vi "Tank Drive.vi"() -> ()   [LabVIEW 2012]
doc: "Tank Drive Example\n\nThis example shows how to implement tank drive and uses two joysticks for input."
uses:
  <vilib>/Rock Robotics/SystemInterfaces/DIO/FPGA_DIOPWMChannel.ctl
  <vilib>/Rock Robotics/WPI/Joystick/WPI_JoystickDeviceEnum.ctl
  <vilib>/Rock Robotics/WPI/Joystick/WPI_JoystickAxis.ctl
  <vilib>/Rock Robotics/WPI/RobotDrive/WPI_RobotDriveOpen2MotorWithJaguar.vi
panel:
  in  "RightStick":T1=enum."USB 2"
  in  "LeftStick":T1
  in  "Left Motor (PWM channel)":T2
  in  "Right Motor (PWM channel)":T2=enum."PWM 2"
  in  "stop":bool
  # "Set these inputs before running."
  # "Wiring Diagram for Digital Sidecar connected to an NI 9403 in slot 4"
  # "Digital Sidecar"
  # "Power\nTerminals"
  # "Motor\nTerminals"
  # "PWM cable"
  # "This shows wiring for a Luminary Micro Jaguar speed controller.  The wiring is similar for a Victor speed controller.  For a Victor, you must also select the appropriate instance of the Motor Open VI on the diagram.  This is only the wiring for the Left Motor.  The Right Motor would be similarly wired to PWM Channel 2."
  # "PWR"
  # "SIG"
  # "(-)"
  # "+V"
  # "10"
  # "9"
  # "8"
  # "7"
  # "6"
  # "5"
  # "4"
  # "3"
  # "2"
  # "1"
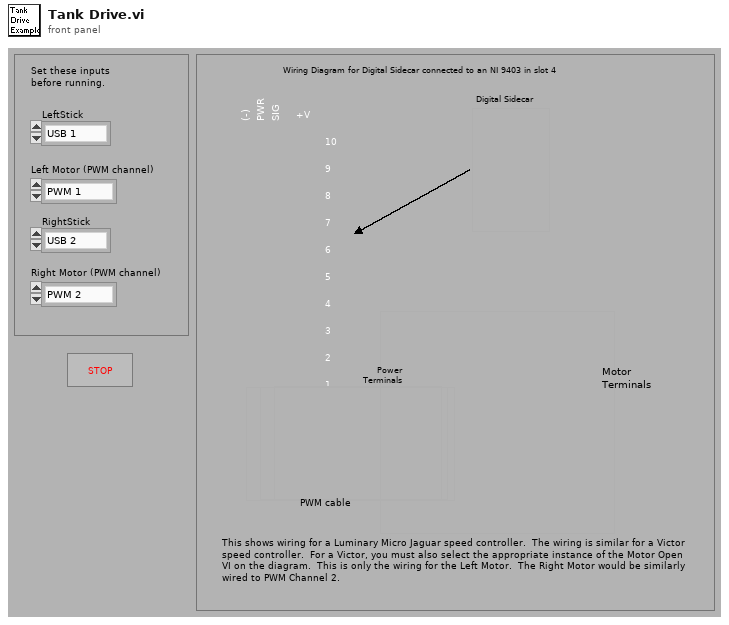
[diagram p1: front panel]
types:
  T1 = typedef "WPI_JoystickDeviceEnum.ctl" = enum16{"USB 1", "USB 2", "USB 3", "USB 4", "Kinect 1", "Kinect 2"}
  T2 = typedef "FPGA_DIOPWMChannel.ctl" = enum8{"PWM 1", "PWM 2", "PWM 3", "PWM 4", "PWM 5", "PWM 6", "PWM 7", "PWM 8", "PWM 9", "PWM 10", "Invalid"}
  T3 = typedef "WPI_JoystickDevRef.ctl" = cluster{"Device":T1}
  T4 = typedef "WPI_RobotDriveDevRef.ctl" = cluster{"DevStatus":errorcluster, "Motors[]":T5[], "Square Inputs":bool, "Max Output":dbl, "Isochronous":bool}
  T5 = typedef "WPI_MotorControlDeviceRef.ctl" = cluster{"DeviceStatus":errorcluster, "Type":enum16{"PWM", "CAN"}, "PWM":cluster{"Digital Module":T6, "PWM Channel":T2, "DeadBand":T7}, "CAN":cluster{"Device Number":u8, "Control Mode":T8, "Semaphore":T9, "Max Vout":dbl}, "Invert":bool, "TransformRef":T10, "InvTransformRef":T10}
  T6 = typedef "FPGA_TypedefDigitalModule.ctl" = enum16{"Digital Module 1", "Digital Module 2"}
  T7 = typedef "WPI_PWMDeadband.ctl" = cluster{"Name":string, "maxPositivePwm":i32, "minPositivePwm":i32, "centerPwm":i32, "maxNegativePwm":i32, "minNegativePwm":i32, "angularRange":u16}
  T8 = typedef "WPI_CANJaguar_ControlMode.ctl" = enum8{"Percent VBus", "Current", "Speed", "Position", "Voltage"}
  T9 = typedef "Semaphore RefNum" = refnum<k1>
  T10 = typedef "WPI_PWMTransform_ConPane.ctl" = refnum<vi>
  T11 = typedef "WPI_JoystickAxis.ctl" = enum16{"Axis 1", "Axis 2", "Axis 3", "Axis 4", "Axis 5", "Axis 6"}
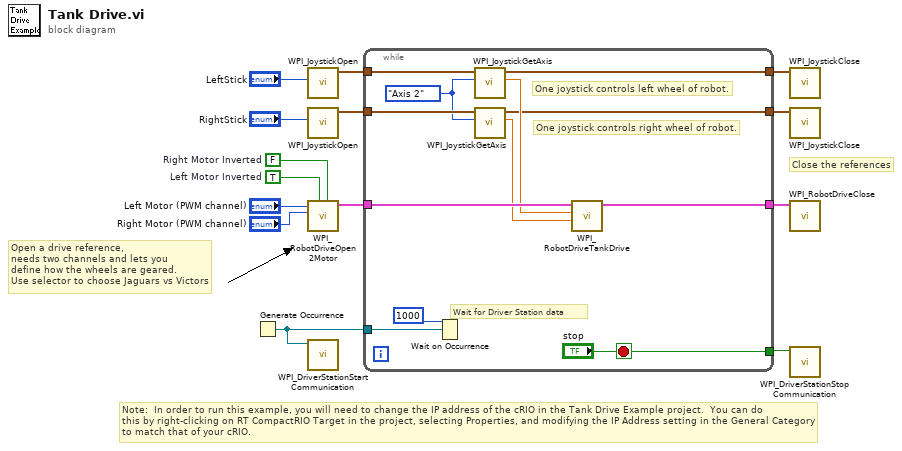
[diagram p0: block diagram]
diagram:
  w7 = FALSE  # Right Motor Inverted
  w8 = TRUE  # Left Motor Inverted
  # "Note:  In order to run this example, you will need to change the IP address of the cRIO in the Tank Drive Example project.  You can do\nthis by right-clicking on RT CompactRIO Target in the project, selecting Properties, and modifying the IP Address setting in the General Category\nto match that of your cRIO."
  # "Close the references"
  # "Open a drive reference,\nneeds two channels and lets you\ndefine how the wheels are geared.\nUse selector to choose Jaguars vs Victors"
  n1 = Generate Occurrence() -> (w10:refnum<k4>)
  n2 = call <vilib>:"WPI_JoystickOpen.vi"("JoystickDevice"="LeftStick") -> ("JoystickDevRef"=w3:T3)  [unwired: 10 out]
  n3 = call <vilib>:"WPI_JoystickOpen.vi"("JoystickDevice"="RightStick") -> ("JoystickDevRef"=w4:T3)  [unwired: 10 out]
  n4 = call-poly <vilib>:"WPI_RobotDriveOpen2Motor.vi"("Right Motor Inverted"=w7, "Left Motor Inverted"=w8, "Right Motor"="Right Motor (PWM channel)", "Left Motor"="Left Motor (PWM channel)") -> ("RobotDriveDevRef"=w12:T4)  [unwired: 1 in, 6 out]
  n5 = call <vilib>:"WPI_DriverStationStart Communication.vi"("occurrence"=w10) -> ()  [unwired: 11 out]
  n6 = while {
    tunnel: w12 -> [w19]
    tunnel: [w20] -> w11
    tunnel: w10 -> [w26]
    tunnel: ["stop"] -> w9
    tunnel: w4 -> [w23]
    tunnel: w3 -> [w22]
    tunnel: [w16] -> w2
    tunnel: [w15] -> w1
    stop <- "stop" stop-if-true
    w21 = WPI_JoystickAxis."Axis 2" ("Axis")
    # "Wait for Driver Station data"
    # "One joystick controls right wheel of robot."
    # "One joystick controls left wheel of robot."
    n7 = Wait on Occurrence(2:w26, 3:1000 ("ms timeout (-1)")) -> ()  [unwired: 2 out]
    n8 = call <vilib>:"WPI_JoystickGetAxis.vi"("Axis"=w21, "JoystickDevRef"=w22) -> ("Value"=w17:dbl, "JoystickDevRef"=w16:T3)  [unwired: 8 out]
    n9 = call <vilib>:"WPI_JoystickGetAxis.vi"("Axis"=w21, "JoystickDevRef"=w23) -> ("Value"=w18:dbl, "JoystickDevRef"=w15:T3)  [unwired: 8 out]
    n10 = call <vilib>:"WPI_RobotDriveTankDrive.vi"("Right axis value"=w18, "Left axis value"=w17, "RobotDriveDevRef"=w19) -> ("RobotDriveDevRef"=w20:T4)  [unwired: 1 in, 7 out]
  }
  n11 = call <vilib>:"WPI_JoystickClose.vi"("JoystickDevRef"=w2) -> ()  [unwired: 11 out]
  n12 = call <vilib>:"WPI_JoystickClose.vi"("JoystickDevRef"=w1) -> ()  [unwired: 11 out]
  n13 = call <vilib>:"WPI_RobotDriveClose.vi"("RobotDriveDevRef"=w11) -> ()  [unwired: 1 in, 10 out]
  n14 = call <vilib>:"WPI_DriverStationStop Communication.vi"("StopCommunication"=w9) -> ()  [unwired: 1 in, 10 out]
